vi "testLatency.vi"() -> ()   [LabVIEW 2017]
uses:
  Adder/Adder0/Adder0.lvclass
  C:/PowerElectronicControl/NonreentrantSinglePoint/dev/Adder/Adder.lvclass
  Subtractor/Subtractor0/Subtractor0.lvclass
  C:/PowerElectronicControl/NonreentrantSinglePoint/dev/Subtractor/Subtractor.lvclass
  Multiplier/Multiply0/Multiplier0.lvclass
  C:/PowerElectronicControl/NonreentrantSinglePoint/dev/Multiplier/Multiplier.lvclass
  Adder/Adder.lvclass
  Multiplier/Multiplier.lvclass
  Subtractor/Subtractor.lvclass
  Adder/Adder1/Adder1.lvclass
  Multiplier/Multiply1/Multiplier1.lvclass
  <vilib>/rvi/Emulation/niFpgaGetClockAttributes.vi
  <vilib>/rvi/Emulation/niFpgaSctlEmulationGetInTimedLoop.vi
  <vilib>/rvi/Emulation/niFpgaEmulationReportErrorSimple.vi
  <vilib>/rvi/Emulation/niFpgaCriticalErrorInLSC.vi
panel:
  out "alpha 2":sgl
  out "beta 2":sgl
  in  "A 2":sgl
  in  "B 2":sgl
  in  "C 2":sgl
  out "alpha":sgl
  out "beta":sgl
  in  "A":sgl
  in  "B":sgl
  in  "C":sgl
  out "rate":u32
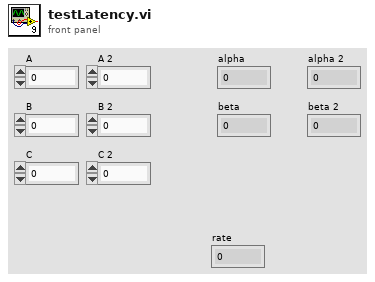
[diagram p1: front panel]
types:
  T1 = cluster{"Adder":refnum<class "Adder.lvclass">, "Multiplier":refnum<class "Multiplier.lvclass">, "Subtractor":refnum<class "Subtractor.lvclass">}
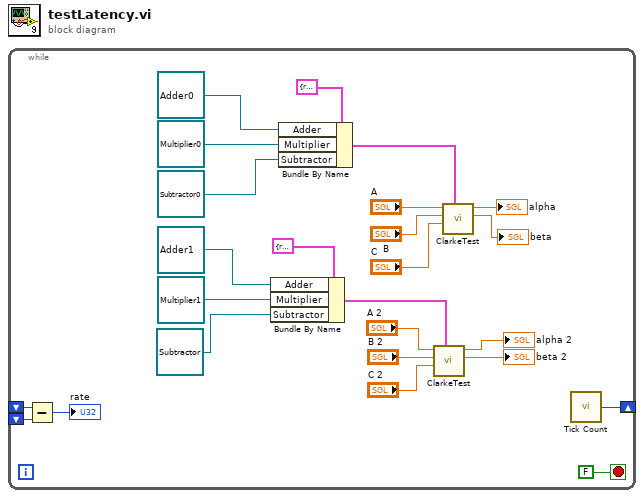
[diagram p0: block diagram]
diagram:
  n1 = while {
    shift-right: [w24] -> _
    shift-left: _ -> [w22]
    shift-left: _ -> [w23]
    stop <- FALSE stop-if-true
    n2 = Subtract(x=w22, y=w23) -> (x-y=→"rate":u32)
    n3 = Bundle By Name(cluster=T1 {"Adder"=refnum, "Multiplier"=refnum, "Subtractor"=refnum} ("Resources"), "Adder"=refnum<class "Adder1.lvclass"> refnum ("Adder1.lvclass"), "Multiplier"=refnum<class "Multiplier1.lvclass"> refnum ("Multiplier1.lvclass"), "Subtractor"=refnum<class "Subtractor.lvclass"> refnum ("Subtractor.lvclass")) -> (w5:T1)
    n4 = Bundle By Name(cluster=T1 {"Adder"=refnum, "Multiplier"=refnum, "Subtractor"=refnum} ("Resources"), "Adder"=refnum<class "Adder0.lvclass"> refnum ("Adder0.lvclass"), "Multiplier"=refnum<class "Multiplier0.lvclass"> refnum ("Multiplier0.lvclass"), "Subtractor"=refnum<class "Subtractor0.lvclass"> refnum ("Subtractor0.lvclass")) -> (w17:T1)
    n5 = call "ClarkeTest.vi"("Resources"=w5, "C"="C 2", "B"="B 2", "A"="A 2") -> ("beta"=→"beta 2":sgl, "alpha"=→"alpha 2":sgl)  [unwired: 6 in]
    n6 = call "ClarkeTest.vi"("Resources"=w17, "C"="C", "B"="B", "A"="A") -> ("beta"=→"beta":sgl, "alpha"=→"alpha":sgl)  [unwired: 6 in]
    n7 = call "Tick Count"() -> ("Tick Count(Ticks)"=w24:u32)
  }
